vi "Get_Values_From_JSON.vi"() -> ()   [LabVIEW 2019]
panel:
  out "value":T1
  out "text":string
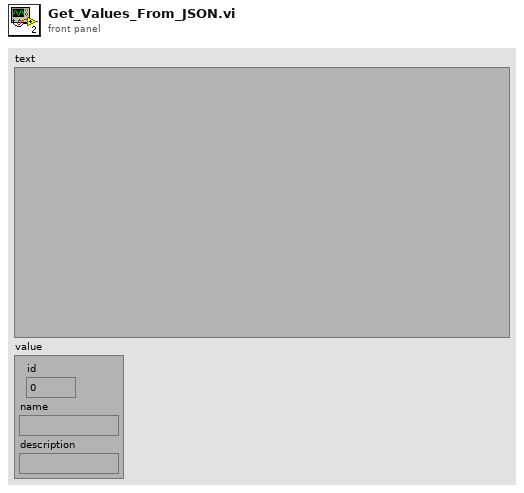
[diagram p1: front panel]
types:
  T1 = cluster{"id":i32, "name":string, "description":string}
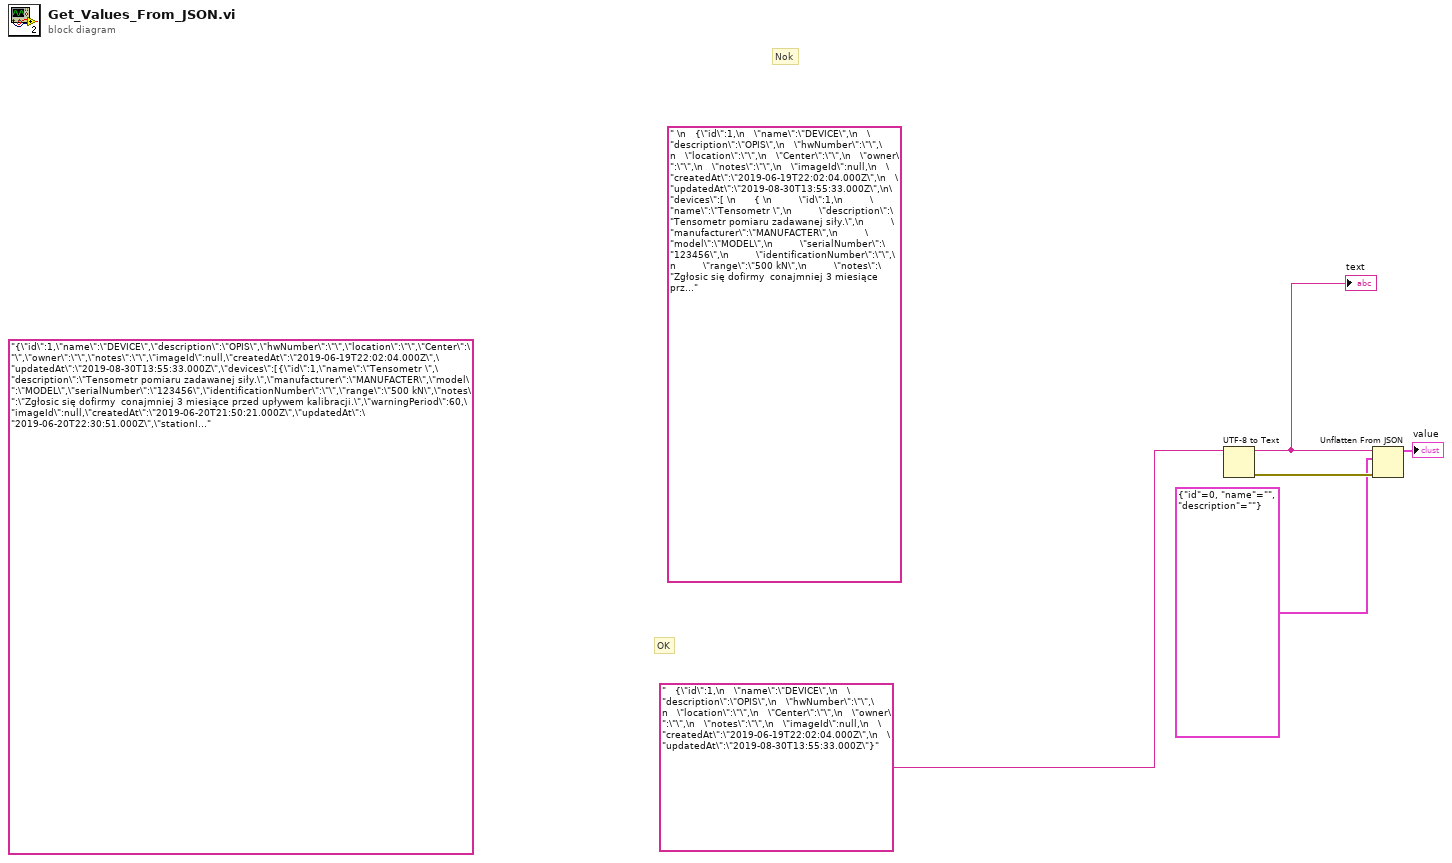
[diagram p0: block diagram]
diagram:
  (unwired) " \n   {\"id\":1,\n   \"name\":\"DEVICE\",\n   \"description\":\"OPIS\",\n   \"hwNumber\":\"\",\n   \"location\":\"\",\n   \"Center\":\"\",\n   \"owner\":\"\",\n   \"notes\":\"\",\n   \"imageId\":null,\n   \"createdAt\":\"2019-06-19T22:02:04.000Z\",\n   \"updatedAt\":\"2019-08-30T13:55:33.000Z\",\n\"devices\":[ \n      { \n         \"id\":1,\n         \"name\":\"Tensometr \",\n         \"description\":\"Tensometr pomiaru zadawanej siły.\",\n         \"manufacturer\":\"MANUFACTER\",\n         \"model\":\"MODEL\",\n         \"serialNumber\":\"123456\",\n         \"identificationNumber\":\"\",\n         \"range\":\"500 kN\",\n         \"notes\":\"Zgłosic się dofirmy  conajmniej 3 miesiące przed upływem kalibracji.\",\n         \"warningPeriod\":60,\n         \"imageId\":null,\n         \"createdAt\":\"2019-06-20T21:50:21.000Z\",\n         \"updatedAt\":\"2019-06-20T22:30:51.000Z\",\n         \"stationId\":1,\n         \"calibration\":{ \n            \"id\":1,\n            \"calibrator\":\"dddffg\",\n            \"date\":\"2019-05-02T00:00:00.000Z\",\n            \"endDate\":\"2020-05-02T00:00:00.000Z\",\n            \"notes\":\"\",\n            \"createdAt\":\"2019-06-20T21:58:21.000Z\",\n            \"updatedAt\":\"2019-06-20T21:58:21.000Z\",\n            \"deviceId\":1,\n            \"userId\":2,\n            \"daysToExpiration\":236.33505163194442,\n            \"daysToWarning\":176.33505163194442,\n            \"status\":\"valid\"\n         }}\n      ]\n}" ("utf-8 text")
  (unwired) "{\"id\":1,\"name\":\"DEVICE\",\"description\":\"OPIS\",\"hwNumber\":\"\",\"location\":\"\",\"Center\":\"\",\"owner\":\"\",\"notes\":\"\",\"imageId\":null,\"createdAt\":\"2019-06-19T22:02:04.000Z\",\"updatedAt\":\"2019-08-30T13:55:33.000Z\",\"devices\":[{\"id\":1,\"name\":\"Tensometr \",\"description\":\"Tensometr pomiaru zadawanej siły.\",\"manufacturer\":\"MANUFACTER\",\"model\":\"MODEL\",\"serialNumber\":\"123456\",\"identificationNumber\":\"\",\"range\":\"500 kN\",\"notes\":\"Zgłosic się dofirmy  conajmniej 3 miesiące przed upływem kalibracji.\",\"warningPeriod\":60,\"imageId\":null,\"createdAt\":\"2019-06-20T21:50:21.000Z\",\"updatedAt\":\"2019-06-20T22:30:51.000Z\",\"stationId\":1,\"calibration\":{\"id\":1,\"calibrator\":\"dddffg\",\"date\":\"2019-05-02T00:00:00.000Z\",\"endDate\":\"2020-05-02T00:00:00.000Z\",\"notes\":\"\",\"createdAt\":\"2019-06-20T21:58:21.000Z\",\"updatedAt\":\"2019-06-20T21:58:21.000Z\",\"deviceId\":1,\"userId\":2,\"daysToExpiration\":236.33505163194442,\"daysToWarning\":176.33505163194442,\"status\":\"valid\"}},{\"id\":2,\"name\":\"Ten\",\"description\":\"mocownik .\",\"manufacturer\":\"fgwr\",\"model\":\"K-11\",\"serialNumber\":\"184009\",\"identificationNumber\":\"\",\"range\":\"10  kN \",\"notes\":\"Poyhyhy.\",\"warningPeriod\":30,\"imageId\":null,\"createdAt\":\"2019-06-20T22:03:26.000Z\",\"updatedAt\":\"2019-06-20T22:03:26.000Z\",\"stationId\":1,\"calibration\":{\"id\":2,\"calibrator\":\"vvvvv\",\"date\":\"2019-05-02T00:00:00.000Z\",\"endDate\":\"2020-05-02T00:00:00.000Z\",\"notes\":\"\",\"createdAt\":\"2019-06-20T22:04:15.000Z\",\"updatedAt\":\"2019-06-20T22:04:15.000Z\",\"deviceId\":2,\"userId\":2,\"daysToExpiration\":236.33505156249998,\"daysToWarning\":206.33505156249998,\"status\":\"valid\"}},{\"id\":3,\"name\":\"fff/ggg\",\"description\":\"Cdhththththdthdi , odthdthdthtp .\",\"manufacturer\":\"hjgkg.\",\"model\":\"\",\"serialNumber\":\"hhh400419001 , \",\"identificationNumber\":\"\",\"range\":\"\",\"notes\":\"\",\"warningPeriod\":30,\"imageId\":null,\"createdAt\":\"2019-06-21T18:28:30.000Z\",\"updatedAt\":\"2019-06-21T18:56:02.000Z\",\"stationId\":1,\"calibration\":{\"id\":3,\"calibrator\":\"\",\"date\":\"2019-05-07T00:00:00.000Z\",\"endDate\":\"2020-05-07T00:00:00.000Z\",\"notes\":\"\",\"createdAt\":\"2019-06-21T18:33:50.000Z\",\"updatedAt\":\"2019-06-21T18:40:37.000Z\",\"deviceId\":3,\"userId\":2,\"daysToExpiration\":241.33505150462963,\"daysToWarning\":211.33505150462963,\"status\":\"valid\"}},{\"id\":4,\"name\":\"Qdfjdjy6\",\"description\":\"Adafgbfgbu \\fbgbfgb\\\".\",\"manufacturer\":\"ggkjl o.o.\",\"model\":\"Qdyjyj6  SN\",\"serialNumber\":\"Qfgbfgb4\",\"identificationNumber\":\"\",\"range\":\"\",\"notes\":\"\",\"warningPeriod\":30,\"imageId\":null,\"createdAt\":\"2019-06-21T18:39:11.000Z\",\"updatedAt\":\"2019-06-21T18:39:11.000Z\",\"stationId\":1,\"calibration\":{\"id\":4,\"calibrator\":\"\",\"date\":\"2019-04-19T00:00:00.000Z\",\"endDate\":\"2020-04-19T00:00:00.000Z\",\"notes\":\"\",\"createdAt\":\"2019-06-21T18:39:40.000Z\",\"updatedAt\":\"2019-06-21T18:39:40.000Z\",\"deviceId\":4,\"userId\":2,\"daysToExpiration\":223.33505144675925,\"daysToWarning\":193.33505144675925,\"status\":\"valid\"}}]}" ("body 2")
  # "Nok"
  # "OK"
  n1 = UTF-8 to Text(11:"   {\"id\":1,\n   \"name\":\"DEVICE\",\n   \"description\":\"OPIS\",\n   \"hwNumber\":\"\",\n   \"location\":\"\",\n   \"Center\":\"\",\n   \"owner\":\"\",\n   \"notes\":\"\",\n   \"imageId\":null,\n   \"createdAt\":\"2019-06-19T22:02:04.000Z\",\n   \"updatedAt\":\"2019-08-30T13:55:33.000Z\"}" ("utf-8 text")) -> (0:w4:errorcluster, 3:w5:string)  [unwired: 2 in]
  "text" <- w5
  n2 = Unflatten From JSON(JSON string=w5, type and defaults=T1 {"id"=0, "name"="", "description"=""}, error in (no error)=w4) -> (value=→"value":T1)  [unwired: 4 in, 1 out]
